vi "getItemsRefs.vi"(8 "error in (no error)":errorcluster, 11 "reference in":refnum<class "Items Controller.lvclass">) -> (0 "error out":errorcluster, 2 "itemsRef":T1, 3 "reference out":refnum<class "Items Controller.lvclass">)   [LabVIEW 2014, in "Items Controller.lvclass"]
uses:
  Items Controller.lvclass
  APP/checkIN_class/checkIN.lvclass
  APP/checkOUT_class/checkOUT.lvclass
  APP/item_class/item.lvclass
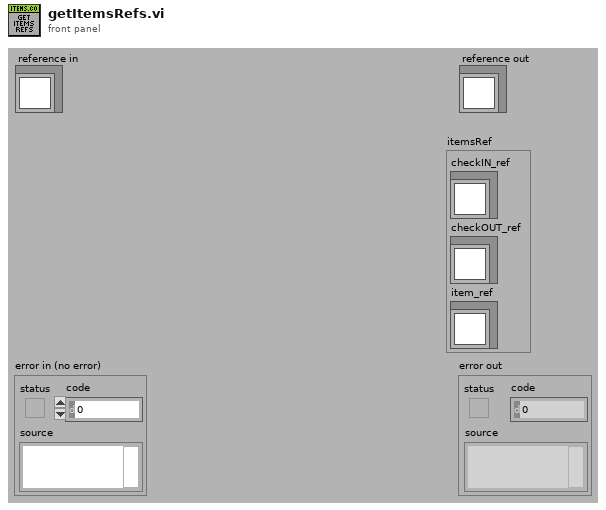
[diagram p1: front panel]
types:
  T1 = cluster{"checkIN_ref":refnum<class "checkIN.lvclass">, "checkOUT_ref":refnum<class "checkOUT.lvclass">, "item_ref":refnum<class "item.lvclass">}
  T2 = typedef "Items Controller.lvclass/ObjectAttributesRef.ctl" = refnum<data-value>
  T3 = typedef "Items Controller.lvclass/ObjectAttributes.ctl" = cluster{"MyAttribute":dbl, "data":string[][][], "file_controller_ref":refnum<class "File Controller.lvclass">, "checkIN_ref":refnum<class "checkIN.lvclass">, "checkOUT_ref":refnum<class "checkOUT.lvclass">, "item_ref":refnum<class "item.lvclass">}
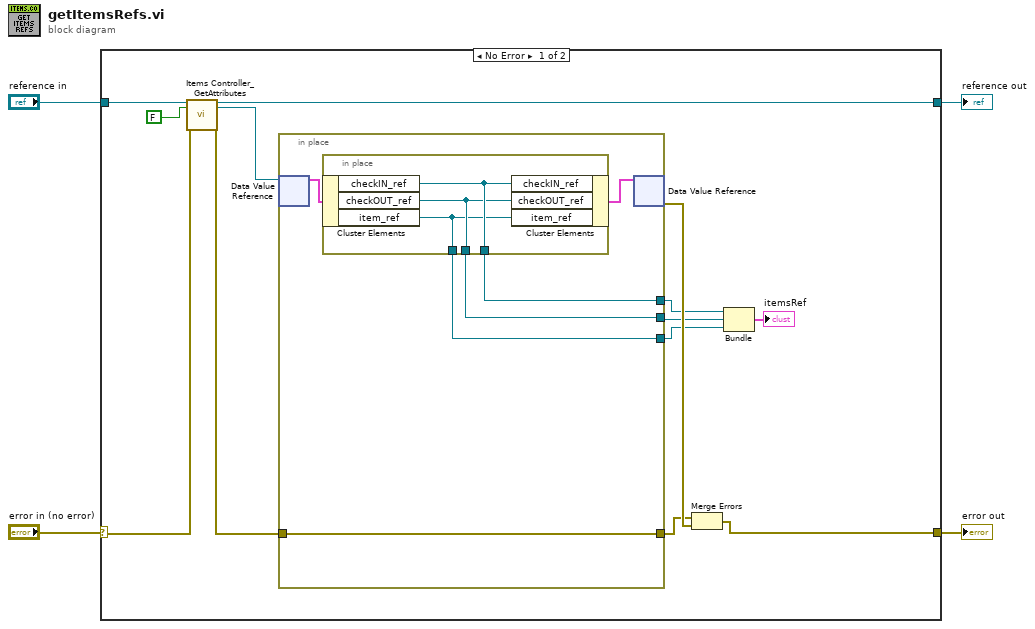
[diagram p0: block diagram]
diagram:
  n1 = case shown="No Error" "error in (no error)" {
    selector: "error in (no error)" -> [w12 w28]
    tunnel: [w17 w28] -> w3
    tunnel: [w10 w27] -> w1
    tunnel: "reference in" -> [w14 w27]
    frame No Error {
      n2 = call "Items Controller_GetAttributes.vi"("reference in"=w14, "return data? (T)"=FALSE, "error in (no error)"=w12) -> ("reference out"=w10:refnum<class "Items Controller.lvclass">, "attributes ref"=w9:T2, "error out"=w11:errorcluster)  [unwired: 13 in, 1 out]
      n3 = in-place {
        in-place-border: w11 -> [w21]
        in-place-border: [w21] -> w15
        in-place-border: [w20] -> w8
        in-place-border: [w19] -> w7
        in-place-border: [w18] -> w6
        n4 = in-place-dvr #1(w9) -> (w22:T3)  [unwired: 1 out]
        n5 = in-place {
          in-place-border: [w26] -> w20
          in-place-border: [w25] -> w19
          in-place-border: [w24] -> w18
          n6 = in-place-cluster #2(w22) -> ("checkIN_ref"=w26:refnum<class "checkIN.lvclass">, "checkOUT_ref"=w25:refnum<class "checkOUT.lvclass">, "item_ref"=w24:refnum<class "item.lvclass">)
          n7 = in-place-cluster #2("checkIN_ref"=w26, "checkOUT_ref"=w25, "item_ref"=w24) -> (w23:T3)
        }
        n8 = in-place-dvr #1(w23) -> (w16:errorcluster)  [unwired: 1 out]
      }
      n9 = Merge Errors(w15, w16) -> (w17:errorcluster)
      n10 = Bundle("checkIN_ref"=w8, "checkOUT_ref"=w7, "item_ref"=w6) -> (→"itemsRef":T1)  [unwired: 1 in]
    }
    frame Error {
    }
  }
  "error out" <- w3
  "reference out" <- w1
